vi "LS Data Global.vi"(2 "Write(T)/Read(F)":bool, 7 "LS Cluster In":T1) -> (8 "LS Cluster Out":T1)   [LabVIEW 2013]
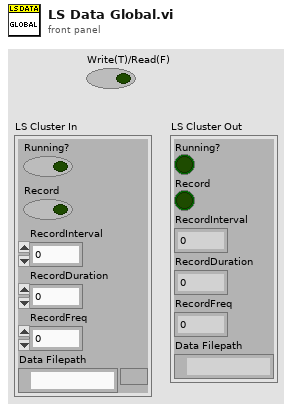
[diagram p1: front panel]
types:
  T1 = cluster{"Running?":bool, "Record":bool, "RecordInterval":i32, "RecordDuration":i32, "RecordFreq":i32, "Data Filepath":path}
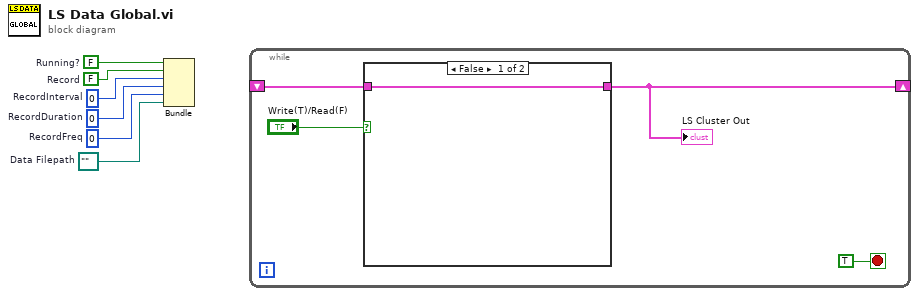
[diagram p0: block diagram]
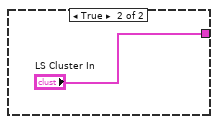
[diagram p2: hidden frame]
diagram:
  w1 = path ""  # Data Filepath
  w2 = 0  # RecordFreq
  w3 = 0  # RecordDuration
  w4 = 0  # RecordInterval
  w5 = FALSE  # Record
  w6 = FALSE  # Running?
  n1 = Bundle("Running?"=w6, "Record"=w5, "RecordInterval"=w4, "RecordDuration"=w3, "RecordFreq"=w2, "Data Filepath"=w1) -> ()  [unwired: 1 in, 1 out]
  n2 = while {
    shift-right: [w7] -> _
    shift-left: _ -> [w9]
    stop <- TRUE stop-if-true
    n3 = case shown="False" "Write(T)/Read(F)" {
      tunnel: w9 -> [w11 _]
      tunnel: [w11 "LS Cluster In"] -> w7
      frame False {
      }
      frame True {
      }
    }
    "LS Cluster Out" <- w7
  }
